vi "ExSubInitCamPulser.vi"(3 "error in (no error)":errorcluster, 4 "Camera Information":T1={"acquire focus mode"=1, "Exposure"=0.0, "Number of Images"=1, "Software accumulation"=1} {"Software accumulation" min=1; "Number of Images" min=1; "Exposure" format="%.2f"; "acquire focus mode" min=1 max=4 step=1}, 5 "Pulser Handle":u32, 6 "Camera Handle":u32) -> (0 "error out":errorcluster, 1 "Pulser Handle":u32, 2 "Camera Handle":u32)   [LabVIEW 2010]
panel:
  # "ExSubInitCamPulser:\nThis Sub VI initializes the camera and \nPulser hardware."
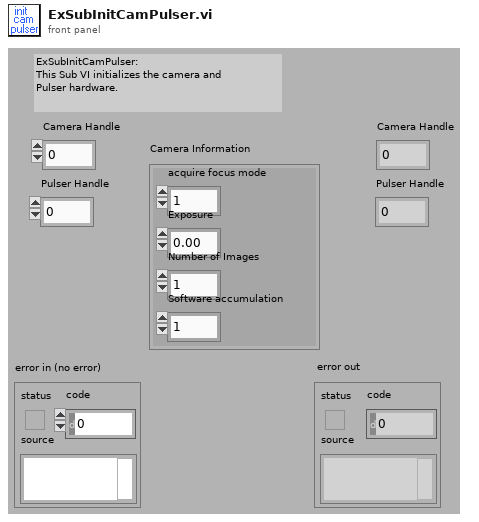
[diagram p1: front panel]
types:
  T1 = cluster{"acquire focus mode":u32, "Exposure":dbl, "Number of Images":u32, "Software accumulation":u32}
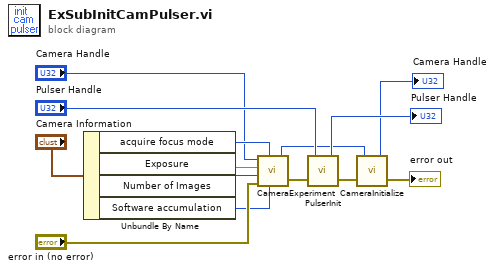
[diagram p0: block diagram]
diagram:
  n1 = Unbundle By Name("Camera Information") -> ("acquire focus mode"=w6:u32, "Exposure"=w5:dbl, "Number of Images"=w4:u32, "Software accumulation"=w3:u32)
  n2 = call <userlib>:"CameraExperiment.vi"("Number of Accumulations"=w3, "Acquire / Focus Flag"=w6, "error in"="error in (no error)", "Number of Images"=w4, "Exposure (sec)"=w5, "Camera Handle"="Camera Handle") -> ("error out"=w11:errorcluster, "Camera Handle"=w7:u32)
  n3 = call <userlib>:"PulserInit.vi"("error in"=w11, "Pulser Handle"="Pulser Handle") -> ("error out"=w14:errorcluster, "Pulser Handle"=→"Pulser Handle":u32)
  n4 = call <userlib>:"CameraInitialize.vi"("error in"=w14, "Camera Handle"=w7) -> ("error out"=→"error out":errorcluster, "Camera Handle"=→"Camera Handle":u32)
